vi "determine_start_block_offset.vi"(7 "force to zero?":bool, 8 "error in (no error)":errorcluster, 11 "DAQmxWriteSignals in":refnum<class "SignalWriterDL090202DAQmx.lvclass">) -> (0 "error out":errorcluster, 3 "DAQmxWriteSignals out":refnum<class "SignalWriterDL090202DAQmx.lvclass">)   [LabVIEW 2010, in "SignalWriterDL090202DAQmx.lvclass"]
uses:
  SignalWriterDL090202DAQmx.lvclass
  GenericSignalWriter/GenericSignalWriter/GenericSignalWriter.lvclass
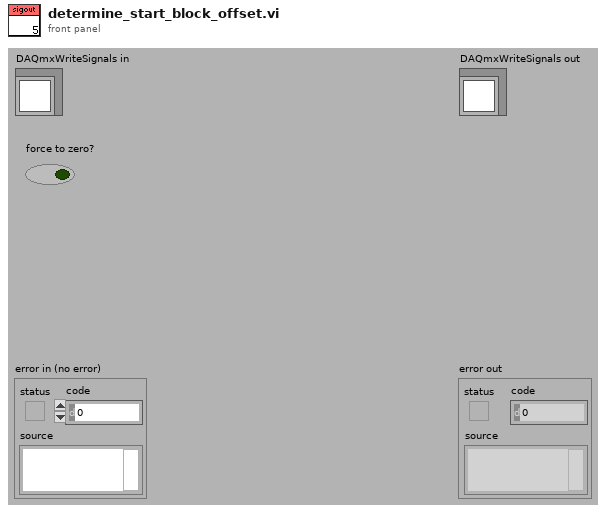
[diagram p1: front panel]
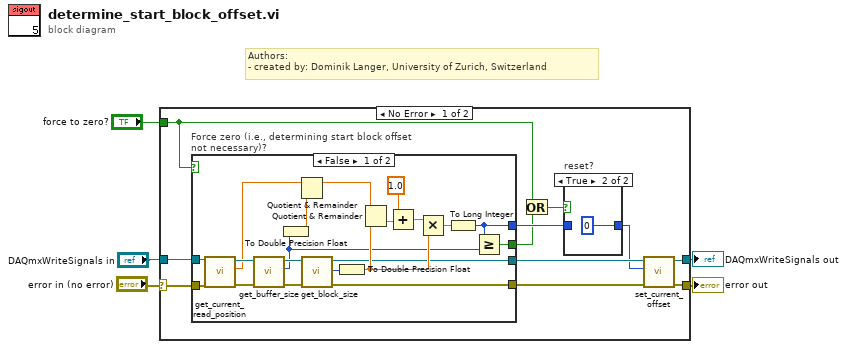
[diagram p0: block diagram]
diagram:
  # "Authors: \n- created by: Dominik Langer, University of Zurich, Switzerland"
  n1 = case shown="No Error" "error in (no error)" {
    selector: "error in (no error)" -> [w16 w42]
    tunnel: [w9 w42] -> w4
    tunnel: [w10 w41] -> w2
    tunnel: "DAQmxWriteSignals in" -> [w15 w41]
    tunnel: "force to zero?" -> [w7 _]
    frame No Error {
      n2 = case "Force zero (i.e., determining start block offset not necessary)?" shown="False" w7 {
        tunnel: w16 -> [w36 w37]
        tunnel: w15 -> [w35 w38]
        tunnel: [w23 w37] -> w14
        tunnel: [w22 w38] -> w13
        tunnel: [w19 _] -> w12
        tunnel: [w18 _] -> w8
        frame False {
          n3 = call "get_current_read_position.vi"("error in (no error)"=w36, "DAQmxWriteSignals in"=w35) -> ("error out"=w29:errorcluster, "current read position"=w27:dbl, "DAQmxWriteSignals out"=w28:refnum<class "SignalWriterDL090202DAQmx.lvclass">)  [unwired: 7 out]
          n4 = call-dynamic "get_buffer_size.vi"("error in (no error)"=w29, "GenericWriteSignals.lvclass in"=w28) -> ("error out"=w26:errorcluster, "buffer size (samples)"=w17:i32, "GenericWriteSignals.lvclass out"=w25:refnum<class "SignalWriterDL090202DAQmx.lvclass">)  [unwired: 7 out]
          n5 = To Double Precision Float(number=w17) -> (double precision float=w20:dbl)
          n6 = Quotient & Remainder(x=w27, y=w20) -> (x-y*floor(x/y)=w24:dbl)  [unwired: 1 out]
          n7 = call "get_block_size.vi"("error in (no error)"=w26, "GenericWriteSignals.lvclass in"=w25) -> ("error out"=w23:errorcluster, "block size"=w34:i32, "GenericWriteSignals.lvclass out"=w22:refnum<class "SignalWriterDL090202DAQmx.lvclass">)  [unwired: 7 out]
          n8 = To Double Precision Float(number=w34) -> (double precision float=w33:dbl)
          n9 = Quotient & Remainder(x=w24, y=w33) -> (floor(x/y)=w32:dbl)  [unwired: 1 out]
          n10 = Add(x=1.0, y=w32) -> (x+y=w31:dbl)
          n11 = Multiply(x=w31, y=w33) -> (x*y=w21:dbl)
          n12 = To Long Integer(number=w21) -> (32bit integer=w19:i32)
          n13 = Greater Or Equal?(x=w19, y=w17) -> (x >= y?=w18:bool)
        }
        frame True {
        }
      }
      n14 = Or(x=w7, y=w8) -> (x .or. y?=w6:bool)
      n15 = case "reset?" shown="True" w6 {
        tunnel: [w39 0] -> w11
        tunnel: w12 -> [w39 _]
        frame False {
        }
        frame True {
        }
      }
      n16 = call-dynamic "set_current_offset.vi"("error in (no error)"=w14, "current offset (samples)"=w11, "GenericWriteSignals.lvclass in"=w13) -> ("error out"=w9:errorcluster, "GenericWriteSignals.lvclass out"=w10:refnum<class "SignalWriterDL090202DAQmx.lvclass">)  [unwired: 7 out]
    }
    frame Error {
    }
  }
  "error out" <- w4
  "DAQmxWriteSignals out" <- w2
